vi "create Behaviour.vi"(8 "error in (no error)":errorcluster caption="Fehler (Eingang, kein Fehler)", 11 "Stoeraussendung Eingang":refnum<class "Stoeraussendung.lvclass"> caption="DNL_LabVIEW Object in") -> (0 "error out":errorcluster caption="Fehler (Ausgang)", 1 "regex":string[](array[string]), 2 "response":bool[](array[boolean]), 3 "Stoeraussendung Ausgang":refnum<class "Stoeraussendung.lvclass"> caption="DNL_LabVIEW Object out")   [LabVIEW 2013, in "Stoeraussendung.lvclass"]
uses:
  Stoeraussendung.lvclass
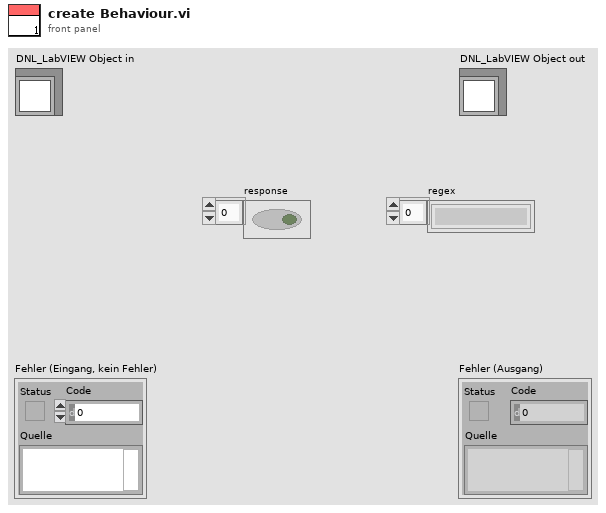
[diagram p1: front panel]
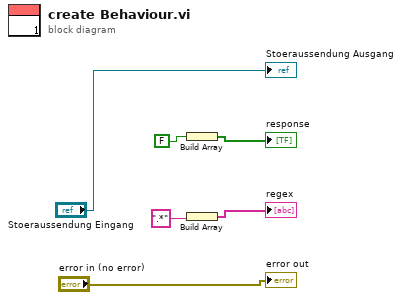
[diagram p0: block diagram]
diagram:
  n1 = Build Array(FALSE) -> (→"response":bool[])
  n2 = Build Array(".*") -> (→"regex":string[])
  "error out" <- "error in (no error)"
  "Stoeraussendung Ausgang" <- "Stoeraussendung Eingang"
